vi "Done Or Abort.vi"(3 "error in (no error)":errorcluster, 5 "MCL State In":refnum<notifier>) -> (0 "error out":errorcluster, 1 "MCL State":T1, 2 "MCL State Out":refnum<notifier>)   [LabVIEW 2009]
uses:
  MCL Done Or Abort.ctl
  MCL States.ctl
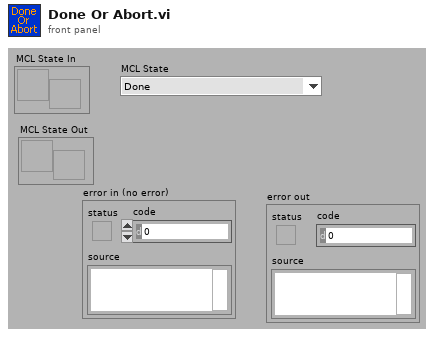
[diagram p1: front panel]
types:
  T1 = typedef "MCL Done Or Abort.ctl" = enum16{"Done", "Abort", "Still Running"}
  T2 = typedef "MCL States.ctl" = enum16{"MCL Idle", "MCL Ramping", "MCL Holding", "MCL Aborting", "MCL Done", "MCL NOP"}
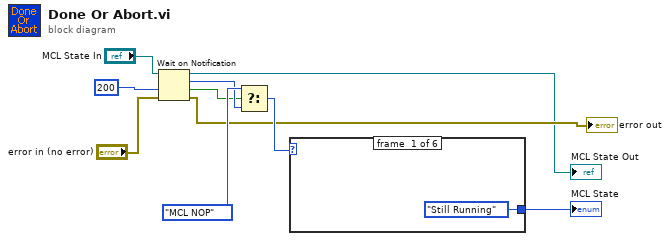
[diagram p0: block diagram]
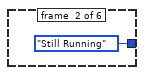
[diagram p2: hidden frame]
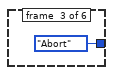
[diagram p3: hidden frame]
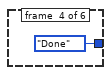
[diagram p4: hidden frame]
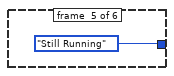
[diagram p5: hidden frame]
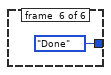
[diagram p6: hidden frame]
diagram:
  n1 = Wait on Notification(notifier="MCL State In", timeout in ms (-1)=200, error in (no error)="error in (no error)") -> (notifier out=→"MCL State Out":refnum<notifier>, notification=w9:T2, timed out?=w8:bool, error out=→"error out":errorcluster)  [unwired: 1 in]
  n2 = Select(t=MCL_States."MCL NOP", s=w8, f=w9) -> (s? t:f=w7:T2)
  n3 = case shown="\"MCL NOP\"" w7 {
    tunnel: [MCL_Done_Or_Abort."Still Running" ("MCL State") MCL_Done_Or_Abort."Still Running" ("MCL State") MCL_Done_Or_Abort."Abort" ("MCL State") MCL_Done_Or_Abort."Done" ("MCL State") MCL_Done_Or_Abort."Still Running" ("MCL State") MCL_Done_Or_Abort."Done" ("MCL State")] -> w1
    frame #0 {
    }
    frame #1 {
    }
    frame #2 {
    }
    frame #3 {
    }
    frame #4 {
    }
    frame #5 {
    }
  }
  "MCL State" <- w1
